vi "BME_DG_GetPCIBusDGInfo.vi"(0 "DG_Number in":i32, 11 "error in (no error)":errorcluster) -> (3 "Master":bool, 4 "DG_Number out":i32, 6 "DG_Product":i32, 8 "SlotNumber":i32, 10 "Bus_Number":i32, 15 "error out":errorcluster)   [LabVIEW 2009, in "POLARIS BME DG.lvlib"]
uses:
  POLARIS BME DG.lvlib
  BME DLL/DelayGenerator.dll
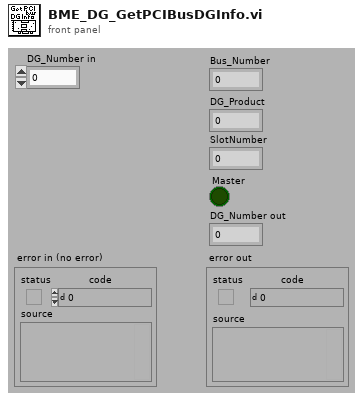
[diagram p1: front panel]
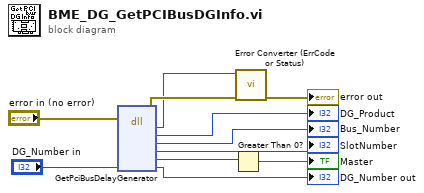
[diagram p0: block diagram]
diagram:
  n1 = dll-call lib="C:/CS Framework/LVSCC/LV2009/GPL/Projects/cs-framework/CSClass/CSPOLARIS/POLARIS BME DG/BME DLL/DelayGenerator.dll" fn="GetPciBusDelayGenerator"(error in="error in (no error)", "DG_Number"="DG_Number in") -> (error out=w3:errorcluster, "return type"=w2:i32, "DG_Product"=→"DG_Product":i32, "Bus_Number"=→"Bus_Number":i32, "SlotNumber"=→"SlotNumber":i32, "Master"=w8:i32, "DG_Number"=→"DG_Number out":i32)  [unwired: 6 in, 1 out]
  n2 = Greater Than 0?(x=w8) -> (x > 0?=→"Master":bool)
  n3 = call "Error Converter (ErrCode or Status).vi"("error in (no error)"=w3, "error code"=w2) -> ("error out"=→"error out":errorcluster)  [unwired: 9 out]
